vi "Run Till Stable1.vi"(11 "output cluster":T1) -> (3 "Stable":bool)   [LabVIEW 2015]
uses:
  Controls/Cal Refs.ctl
  <vilib>/Analysis/baseanly.llb/Mean (DBL).vi
  <vilib>/Analysis/NI_AALBase.lvlib
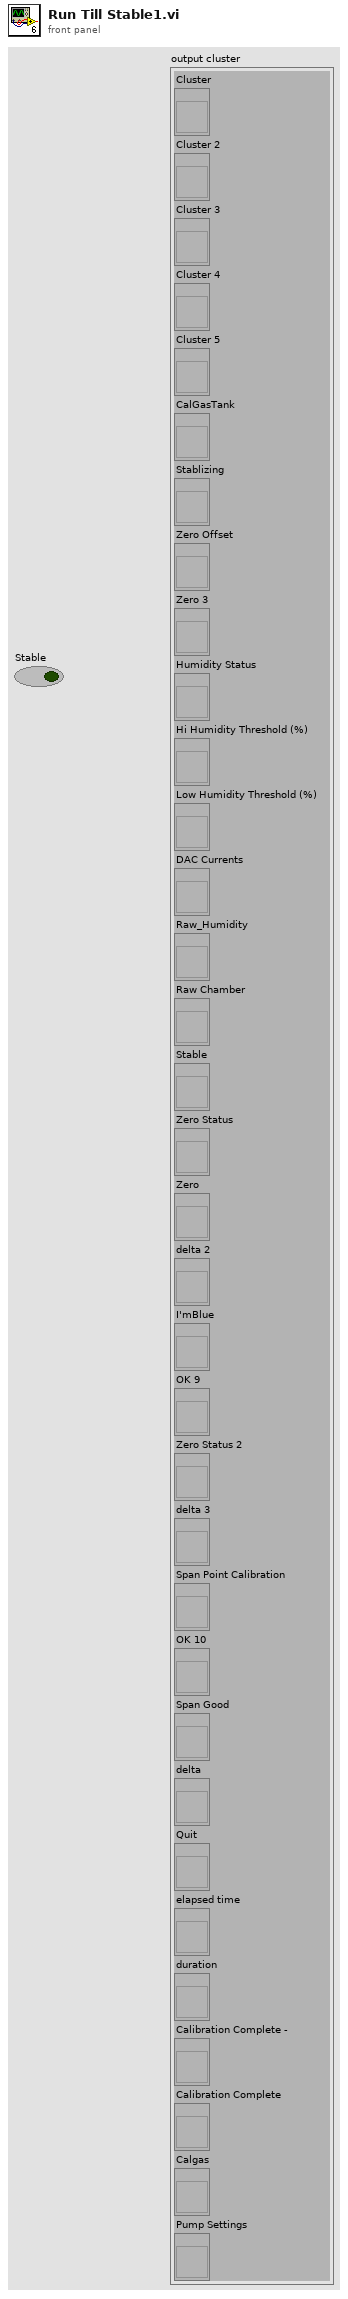
[diagram p1: front panel]
types:
  T1 = typedef "Cal Refs.ctl" = cluster{"Cluster":refnum<vi>, "Cluster 2":refnum<vi>, "Cluster 3":refnum<vi>, "Cluster 4":refnum<vi>, "Cluster 5":refnum<vi>, "CalGasTank":refnum<vi>, "Stablizing":refnum<vi>, "Zero Offset":refnum<vi>, "Zero 3":refnum<vi>, "Humidity Status":refnum<vi>, "Hi Humidity Threshold (%)":refnum<vi>, "Low Humidity Threshold (%)":refnum<vi>, "DAC Currents":refnum<vi>, "Raw_Humidity":refnum<vi>, "Raw Chamber":refnum<vi>, "Stable":refnum<vi>, "Zero Status":refnum<vi>, "Zero":refnum<vi>, "delta 2":refnum<vi>, "I'mBlue":refnum<vi>, "OK 9":refnum<vi>, "Zero Status 2":refnum<vi>, "delta 3":refnum<vi>, "Span Point Calibration":refnum<vi>, "OK 10":refnum<vi>, "Span Good":refnum<vi>, "delta":refnum<vi>, "Quit":refnum<vi>, "elapsed time":refnum<vi>, "duration":refnum<vi>, "Calibration Complete -":refnum<vi>, "Calibration Complete":refnum<vi>, "Calgas":refnum<vi>, "Pump Settings":refnum<vi>}
  T2 = cluster{"Tcal_Chamber":dbl, "Tcal_PCB":dbl, "Tcal_Film":dbl, "Tcal_Humidity":dbl, "Tcal_Det":dbl[], "Cal Gas":dbl, "Reference":dbl}
  T3 = cluster{"CalFile Selected":path, "TYPE":string, "DATE":string, "C0FC2V":dbl[], "C6FC2V":dbl[], "V_0d(target)":dbl[], "V_6d(target)":dbl[], "V_span(target)":dbl[], "CHANNEL":string[], "Status":bool[], "BlueLED 2":bool[], "C2V":u8[], "A":dbl[], "B":dbl[], "C":dbl[], "D":dbl[], "V2C":u8[], "A'":dbl[], "B'":dbl[], "C'":dbl[], "D'":dbl[]}
  T4 = cluster{"CHANNEL 2":string[], "BlueLED":bool[], "V_RA(5mA)":dbl[], "V_RA(15mA)":dbl[], "mI":dbl[], "DAC scale":dbl[]}
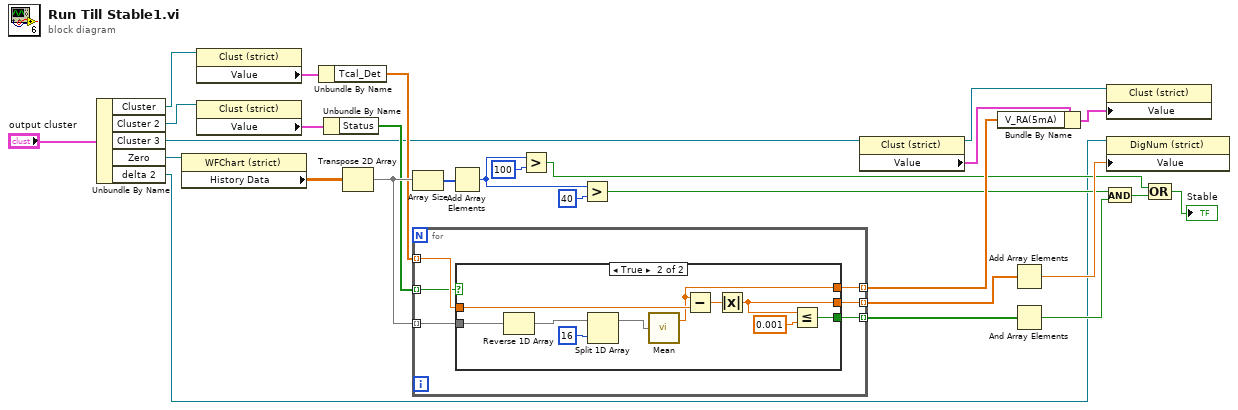
[diagram p0: block diagram]
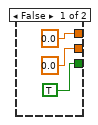
[diagram p2: hidden frame]
diagram:
  n1 = Unbundle By Name("output cluster") -> ("Cluster"=w7:refnum<vi>, "Cluster 2"=w5:refnum<vi>, "Cluster 3"=w3:refnum<vi>, "Zero"=w2:refnum<vi>, "delta 2"=w1:refnum<vi>)
  n2 = property on="Property Node" class="WFChart (strict)"(reference=w2) -> ("History Data"=w15:dbl[][])  [unwired: 1 in, 2 out]
  n3 = property class="Clust (strict)"(reference=w7) -> ("Value"=w8:T2)  [unwired: 1 in, 2 out]
  n4 = property class="Clust (strict)"(reference=w5) -> ("Value"=w9:T3)  [unwired: 1 in, 2 out]
  n5 = Unbundle By Name(w8) -> ("Tcal_Det"=w6:dbl[])
  n6 = Unbundle By Name(w9) -> ("Status"=w4:bool[])
  n7 = Transpose 2D Array(2D array=w15) -> (transposed array=w16:dbl[][])
  n8 = Array Size(array=w16) -> (size(s)=w11:i32[])
  n9 = for {
    tunnel: w16 -> [w34] mode=indexing
    tunnel: w6 -> [w33] mode=indexing
    tunnel: [w32] -> w17 mode=indexing
    tunnel: [w31] -> w28 mode=indexing
    tunnel: [w30] -> w24 mode=indexing
    tunnel: w4 -> [w29] mode=indexing
    n10 = case shown="True" w29 {
      tunnel: w34 -> [_ w42]
      tunnel: w33 -> [_ w41]
      tunnel: [TRUE w40] -> w32
      tunnel: [0.0 ("mean") w39] -> w31
      tunnel: [0.0 w38] -> w30
      frame False {
      }
      frame True {
        n11 = Reverse 1D Array(array=w42) -> (reversed array=w43:dbl[])
        n12 = Split 1D Array(array=w43, index=16) -> (first subarray=w44:dbl[])  [unwired: 1 out]
        n13 = call-poly <vilib>:"Mean.vi"("X"=w44) -> ("mean"=w39:dbl)  [unwired: 1 out]
        n14 = Subtract(x=w39, y=w41) -> (x-y=w46:dbl)
        n15 = Absolute Value(x=w46) -> (abs(x)=w38:dbl)
        n16 = Less Or Equal?(x=w38, y=0.001) -> (x <= y?=w40:bool)
      }
    }
  }
  n17 = Add Array Elements(numeric array=w11) -> (sum=w22:i32)
  n18 = Greater?(x=w22, y=100 ("index")) -> (0:w21:bool)
  n19 = Greater?(x=w22, y=40 ("index")) -> (0:w13:bool)
  n20 = property class="Clust (strict)"(reference=w3) -> (reference out=w25:refnum<vi>, "Value"=w26:T4)  [unwired: 1 in, 1 out]
  n21 = Bundle By Name(cluster=w26, "V_RA(5mA)"=w28) -> (w27:T4)
  n22 = Add Array Elements(numeric array=w24) -> (sum=w23:dbl)
  n23 = And Array Elements(Boolean array=w17) -> (logical AND=w18:bool)
  n24 = And(x=w13, y=w18) -> (x .and. y?=w20:bool)
  n25 = property class="Clust (strict)"(reference=w25, "Value"=w27) -> ()  [unwired: 1 in, 2 out]
  n26 = property class="DigNum (strict)"(reference=w1, "Value"=w23) -> ()  [unwired: 1 in, 2 out]
  n27 = Compound Arithmetic op=OR(w21, w20) -> (→"Stable":bool)
